vi "Plugin - View(XYGraph).vi"() -> ()   [LabVIEW 2016]
uses:
  Library/Queue/old vi/QueueMakeMode.ctl
  GraphSetting/TypeDef/XYData.ctl
  GraphSetting/Dialog/Dialog GraphSetting (XY).vi
  <vilib>/measure/NI_MABase.lvlib
panel:
  in  "パラメータ":string[](array[string])
  out "XYグラフ":cluster{"X":dbl[], "Y":dbl[]}[](graph)
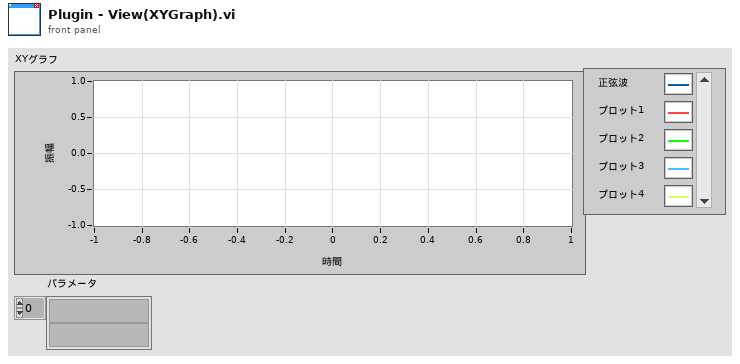
[diagram p1: front panel]
types:
  T1 = typedef "QueueMakeMode.ctl" = enum16{"Create", "Get", "Release", "ReleaseAll"}
  T2 = typedef "XYData.ctl" = cluster{"X":dbl[], "Y":dbl[]}
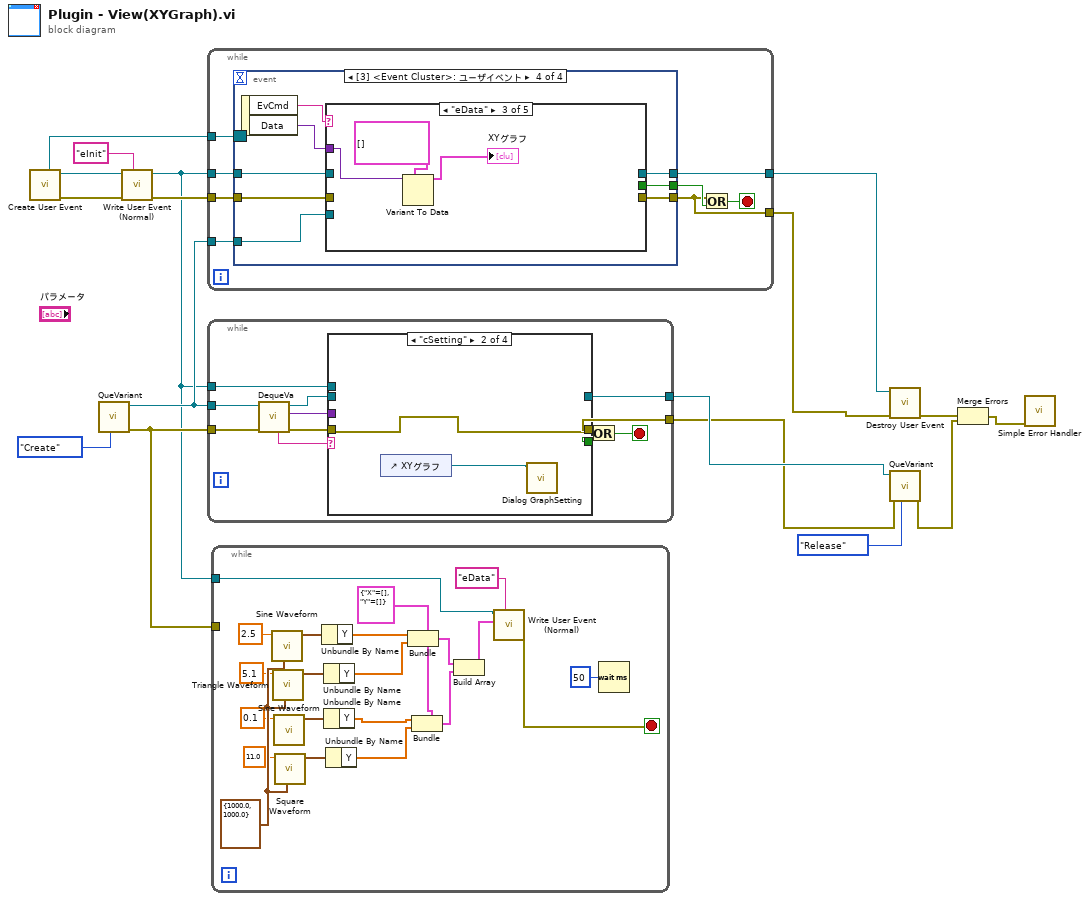
[diagram p0: block diagram]
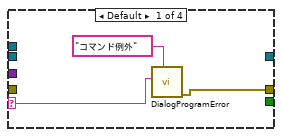
[diagram p2: hidden frame]
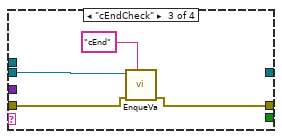
[diagram p3: hidden frame]
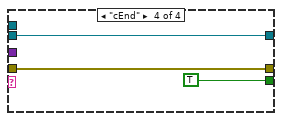
[diagram p4: hidden frame]
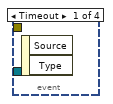
[diagram p5: hidden frame]
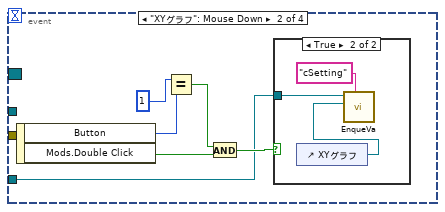
[diagram p6: hidden frame]
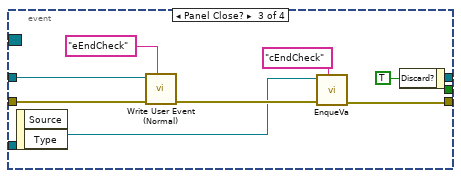
[diagram p8: hidden frame]
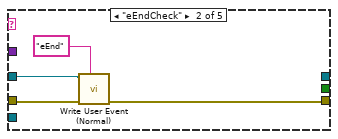
[diagram p10: hidden frame]
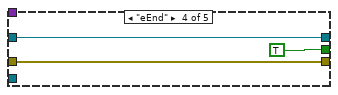
[diagram p11: hidden frame]
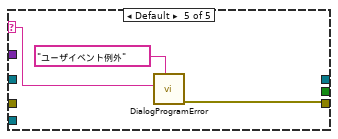
[diagram p12: hidden frame]
diagram:
  n1 = call "Create User Event.vi"() -> ("error out"=w12:errorcluster, "User Event"=w13:refnum<user-event>, "Event Registration Refnum"=w14:refnum<event-registration>)  [unwired: 9 in]
  n2 = call "QueVariant.vi"("MODE(GET)"=QueueMakeMode."Create") -> ("error out"=w2:errorcluster, "queVariant"=w3:refnum<queue>)  [unwired: 9 in]
  n3 = call "Write User Event (Normal).vi"("EvCmd"="eInit", "エラー入力（エラーなし）"=w12, "ユーザイベント入力"=w13) -> ("エラー出力"=w11:errorcluster, "ユーザイベント出力"=w1:refnum<user-event>)  [unwired: 7 in]
  n4 = while {
    tunnel: w11 -> [w21]
    tunnel: w3 -> [w25]
    tunnel: w14 -> [w22]
    tunnel: [w20] -> w9
    tunnel: w1 -> [w19]
    tunnel: [w18] -> w10
    stop <- w23 stop-if-true
    n5 = event shown="[3] <Event Cluster>: ユーザイベント" {
      selector: w22 -> [_ _ _ _]
      dyn-events: _ -> [_ _ _ _]
      timeout: _ -> [_ _ _ _]
      tunnel: [_ _ _ w45] -> w24
      tunnel: w25 -> [_ w26 w36 w48]
      tunnel: [_ _ w37 w46] -> w20
      tunnel: w21 -> [_ _ w41 w47]
      tunnel: w19 -> [_ _ w42 w44]
      tunnel: [_ _ _ w43] -> w18
      event Timeout {
        n6 = event-data() -> ()  [unwired: 1 in, 2 out]
      }
      event "XYグラフ": Mouse Down {
        n7 = event-data() -> ("Button"=w30:u16, "Mods.Double Click"=w28:bool)  [unwired: 1 in]
        n8 = Equal?(x=u16 1 ("ボタン"), y=w30) -> (x = y?=w29:bool)
        n9 = And(x=w29, y=w28) -> (x .and. y?=w27:bool)
        n10 = case shown="TRUE" w27 {
          tunnel: w26 -> [_ w34]
          frame False {
          }
          frame True {
            n11 = control-ref of="XYグラフ"() -> (w32:refnum<vi>)
            n12 = call "EnqueVa.vi"("コマンド"="cSetting", "バリアント"=w32, "queVariant"=w34) -> ()  [unwired: 6 in, 3 out]
          }
        }
      }
      event Panel Close? {
        n13 = event-data() -> ()  [unwired: 1 in, 2 out]
        n14 = call "Write User Event (Normal).vi"("EvCmd"="eEndCheck", "エラー入力（エラーなし）"=w41, "ユーザイベント入力"=w42) -> ("エラー出力"=w38:errorcluster)  [unwired: 7 in, 1 out]
        n15 = call "EnqueVa.vi"("コマンド"="cEndCheck", "エラー入力（エラーなし）"=w38, "queVariant"=w36) -> ("エラー出力"=w37:errorcluster)  [unwired: 6 in, 2 out]
        n16 = event-data("Discard?"=TRUE ("破棄?")) -> ()  [unwired: 1 in, 1 out]
      }
      event User Event {
        n17 = event-data() -> ("EvCmd"=w50:string, "Data"=w49:variant)  [unwired: 1 in]
        n18 = case shown="\"eData\"" w50 {
          selector: w50 -> [_ _ _ _ w62]
          tunnel: w49 -> [_ _ w57 _ _]
          tunnel: w48 -> [_ _ _ _ _]
          tunnel: w47 -> [_ w52 _ w59 _]
          tunnel: [_ w51 _ w59 w61] -> w46
          tunnel: [_ _ _ TRUE _] -> w45
          tunnel: w44 -> [_ w54 _ w60 _]
          tunnel: [_ _ _ w60 _] -> w43
          frame "eInit" {
          }
          frame "eEndCheck" {
            n19 = call "Write User Event (Normal).vi"("EvCmd"="eEnd", "エラー入力（エラーなし）"=w52, "ユーザイベント入力"=w54) -> ("エラー出力"=w51:errorcluster)  [unwired: 7 in, 1 out]
          }
          frame "eData" {
            n20 = Variant To Data(type=T2[] [], Variant=w57) -> (data=→"XYグラフ":T2[])  [unwired: 1 in, 1 out]
          }
          frame "eEnd" {
          }
          frame Default {
            n21 = call "DialogProgramError.vi"("エラー内容"="ユーザイベント例外" ("エラー詳細"), "エラー詳細"=w62) -> ("error out"=w61:errorcluster)  [unwired: 9 in]
          }
        }
      }
    }
    n22 = Or(x=w20, y=w24) -> (x .or. y?=w23:bool)
  }
  n23 = while {
    tunnel: w3 -> [w74]
    tunnel: w2 -> [w73]
    tunnel: w1 -> [w67]
    tunnel: [w66] -> w7
    tunnel: [w64] -> w8
    stop <- w68 stop-if-true
    n24 = call "DequeVa.vi"("エラー入力（エラーなし）"=w73, "queVariant"=w74) -> ("エラー出力"=w70:errorcluster, "バリアント"=w71:variant, "queVariant(copy)"=w65:refnum<queue>, "コマンド"=w72:string)  [unwired: 5 in, 1 out]
    n25 = case shown="\"cSetting\"" w72 {
      selector: w72 -> [w76 _ _ _]
      tunnel: w71 -> [_ _ _ _]
      tunnel: [_ _ _ TRUE] -> w69
      tunnel: [w75 w79 w81 w84] -> w66
      tunnel: w70 -> [_ w79 w82 w84]
      tunnel: w67 -> [_ _ _ _]
      tunnel: w65 -> [_ _ w83 w86]
      tunnel: [_ _ _ w86] -> w64
      frame Default {
        n26 = call "DialogProgramError.vi"("エラー内容"="コマンド例外" ("エラー詳細"), "エラー詳細"=w76) -> ("error out"=w75:errorcluster)  [unwired: 9 in]
      }
      frame "cSetting" {
        n27 = control-ref of="XYグラフ"() -> (w78:refnum<vi>)
        n28 = call-poly "Dialog GraphSetting.vi"("XYグラフref(in)"=w78) -> ()  [unwired: 11 in]
      }
      frame "cEndCheck" {
        n29 = call "EnqueVa.vi"("コマンド"="cEnd", "エラー入力（エラーなし）"=w82, "queVariant"=w83) -> ("エラー出力"=w81:errorcluster)  [unwired: 6 in, 2 out]
      }
      frame "cEnd" {
      }
    }
    n30 = Or(x=w66, y=w69) -> (x .or. y?=w68:bool)
  }
  n31 = while {
    tunnel: w2 -> [_]
    tunnel: w1 -> [w106]
    stop <- w104 stop-if-true
    w93 = T2 {"X"=[], "Y"=[]} ("XYグラグデータ")
    w95 = cluster{"Fs":dbl, "#s":dbl} {"Fs"=1000.0, "#s"=1000.0} ("sampling info")
    n32 = call <vilib>:"Sine Waveform.vi"("sampling info"=w95, "frequency"=2.5) -> ("signal out"=w101:waveform(dbl))  [unwired: 8 in, 1 out]
    n33 = call <vilib>:"Triangle Waveform.vi"("sampling info"=w95, "frequency"=5.1) -> ("signal out"=w103:waveform(dbl))  [unwired: 8 in, 1 out]
    n34 = call <vilib>:"Sine Waveform.vi"("frequency"=0.1) -> ("signal out"=w97:waveform(dbl))  [unwired: 9 in, 1 out]
    n35 = call <vilib>:"Square Waveform.vi"("sampling info"=w95, "frequency"=11.0) -> ("signal out"=w96:waveform(dbl))  [unwired: 8 in, 1 out]
    n36 = Unbundle By Name(w101) -> ("Y"=w102:dbl[])
    n37 = Unbundle By Name(w103) -> ("Y"=w98:dbl[])
    n38 = Unbundle By Name(w97) -> ("Y"=w94:dbl[])
    n39 = Unbundle By Name(w96) -> ("Y"=w92:dbl[])
    n40 = Bundle(cluster=w93, "X"=w102, "Y"=w98) -> (w100:T2)
    n41 = Bundle(cluster=w93, "X"=w94, "Y"=w92) -> (w91:T2)
    n42 = Build Array(w100, w91) -> (w99:T2[])
    n43 = call "Write User Event (Normal).vi"("EvCmd"="eData" ("コマンド"), "データ"=w99, "ユーザイベント入力"=w106) -> ("エラー出力"=w104:errorcluster)  [unwired: 7 in, 1 out]
    n44 = Wait (ms)(milliseconds to wait=u32 50) -> ()  [unwired: 1 out]
  }
  n45 = call "Destroy User Event.vi"("error in (no error)"=w9, "User Event"=w10) -> ("error out"=w6:errorcluster)  [unwired: 9 in]
  n46 = call "QueVariant.vi"("MODE(GET)"=QueueMakeMode."Release", "error in"=w7, "queVariant(in)"=w8) -> ("error out"=w5:errorcluster)  [unwired: 7 in, 1 out]
  n47 = Merge Errors(w6, w5) -> (w4:errorcluster)
  n48 = call <vilib>:"Simple Error Handler.vi"("error in (no error)"=w4) -> ()  [unwired: 4 in, 5 out]
